vi "generator_set_values.vi"(8 "error in (no error)":errorcluster, 9 "Frequency (1000 Hz)":dbl=1000.0 format="%#.6g", 10 "Amplitude (1.0 Vpp)":dbl=1.0 format="%#.4f", 11 "app_data":T1={"Instruments"={"generator"="", "voltment_with_scaner"="", "voltment_without_scaner"=""}, "boc"={"conParam"={"ReadIntParam"=TRUE, "ReadDescrParam"=FALSE, "ReadFloatParam"=TRUE, "debug"=FALSE, "ReadJSON"=FALSE, "IP_address"="192.168.1.216", "N_attempts"=3, "type_con"=enum."TCP", "MB_address"=1, "VISA"="COM1", "connection ID"=refnum, "nameDevices"="", "timeout"=3000, "port"=2000, "type_version"="0F0C0001", "baud_rate"=115200, "VersionControl"=FALSE, "TCP_conn"=FALSE, "WindowSize"=700}, "Param"={"NumParam"={"NTelem"=0, "NInt"=0, "NFloat"=0, "NTable"=0}, "ParamInt"=[], "Telemetry"=[], "Table"=[], "ParamFloat"=[]}}, "boe"={"conParam"={"ReadIntParam"=TRUE, "ReadDescrParam"=FALSE, "ReadFloatParam"=TRUE, "debug"=FALSE, "ReadJSON"=FALSE, "IP_address"="192.168.1.216", "N_attempts"=3, "type_con"=enum."TCP", "MB_address"=1, "VISA"="COM1", "connection ID"=refnum, "nameDevices"="", "timeout"=3000, "port"=2000, "type_version"="03200100", "baud_rate"=115200, "VersionControl"=FALSE, "TCP_conn"=FALSE, "WindowSize"=700}, "Param"={"NumParam"={"NTelem"=0, "NInt"=0, "NFloat"=0, "NTable"=0}, "ParamInt"=[], "Telemetry"=[], "Table"=[], "ParamFloat"=[]}}, "attenuator_tune_koef"=[]}) -> (0 "error out":errorcluster, 3 "output cluster":T1={"Instruments"={"generator"="", "voltment_with_scaner"="", "voltment_without_scaner"=""}, "boc"={"conParam"={"ReadIntParam"=TRUE, "ReadDescrParam"=FALSE, "ReadFloatParam"=TRUE, "debug"=FALSE, "ReadJSON"=TRUE, "IP_address"="192.168.1.216", "N_attempts"=3, "type_con"=enum."TCP", "MB_address"=1, "VISA"="COM1", "connection ID"=refnum, "nameDevices"="", "timeout"=3000, "port"=2000, "type_version"="0F0C0001", "baud_rate"=115200, "VersionControl"=FALSE, "TCP_conn"=FALSE, "WindowSize"=700}, "Param"={"NumParam"={"NTelem"=0, "NInt"=0, "NFloat"=0, "NTable"=0}, "ParamInt"=[], "Telemetry"=[], "Table"=[], "ParamFloat"=[]}}, "boe"={"conParam"={"ReadIntParam"=TRUE, "ReadDescrParam"=FALSE, "ReadFloatParam"=TRUE, "debug"=FALSE, "ReadJSON"=TRUE, "IP_address"="192.168.1.216", "N_attempts"=3, "type_con"=enum."TCP", "MB_address"=1, "VISA"="COM1", "connection ID"=refnum, "nameDevices"="", "timeout"=3000, "port"=2000, "type_version"="0F0C0001", "baud_rate"=115200, "VersionControl"=FALSE, "TCP_conn"=FALSE, "WindowSize"=700}, "Param"={"NumParam"={"NTelem"=0, "NInt"=0, "NFloat"=0, "NTable"=0}, "ParamInt"=[], "Telemetry"=[], "Table"=[], "ParamFloat"=[]}}, "attenuator_tune_koef"=[]})   [LabVIEW 2017]
uses:
  controls/app_data.ctl
  controls/instruments.ctl
  Unicorn Labview Library/Control/unicorn_Param.ctl
  Unicorn Labview Library/Control/unicorn_conn.ctl
  Unicorn Labview Library/Control/unicorn_JSON.ctl
  Unicorn Labview Library/Control/unicorn_ParamInt.ctl
  Unicorn Labview Library/Control/unicorn_Telemetry.ctl
  Unicorn Labview Library/Control/unicorn_Table.ctl
  Unicorn Labview Library/Control/unicorn_ParamFloat.ctl
  <instrlib>/Siglent SDG X Series/Siglent SDG X Series.lvlib
  Unicorn Labview Library/Unicorn Library.lvlib
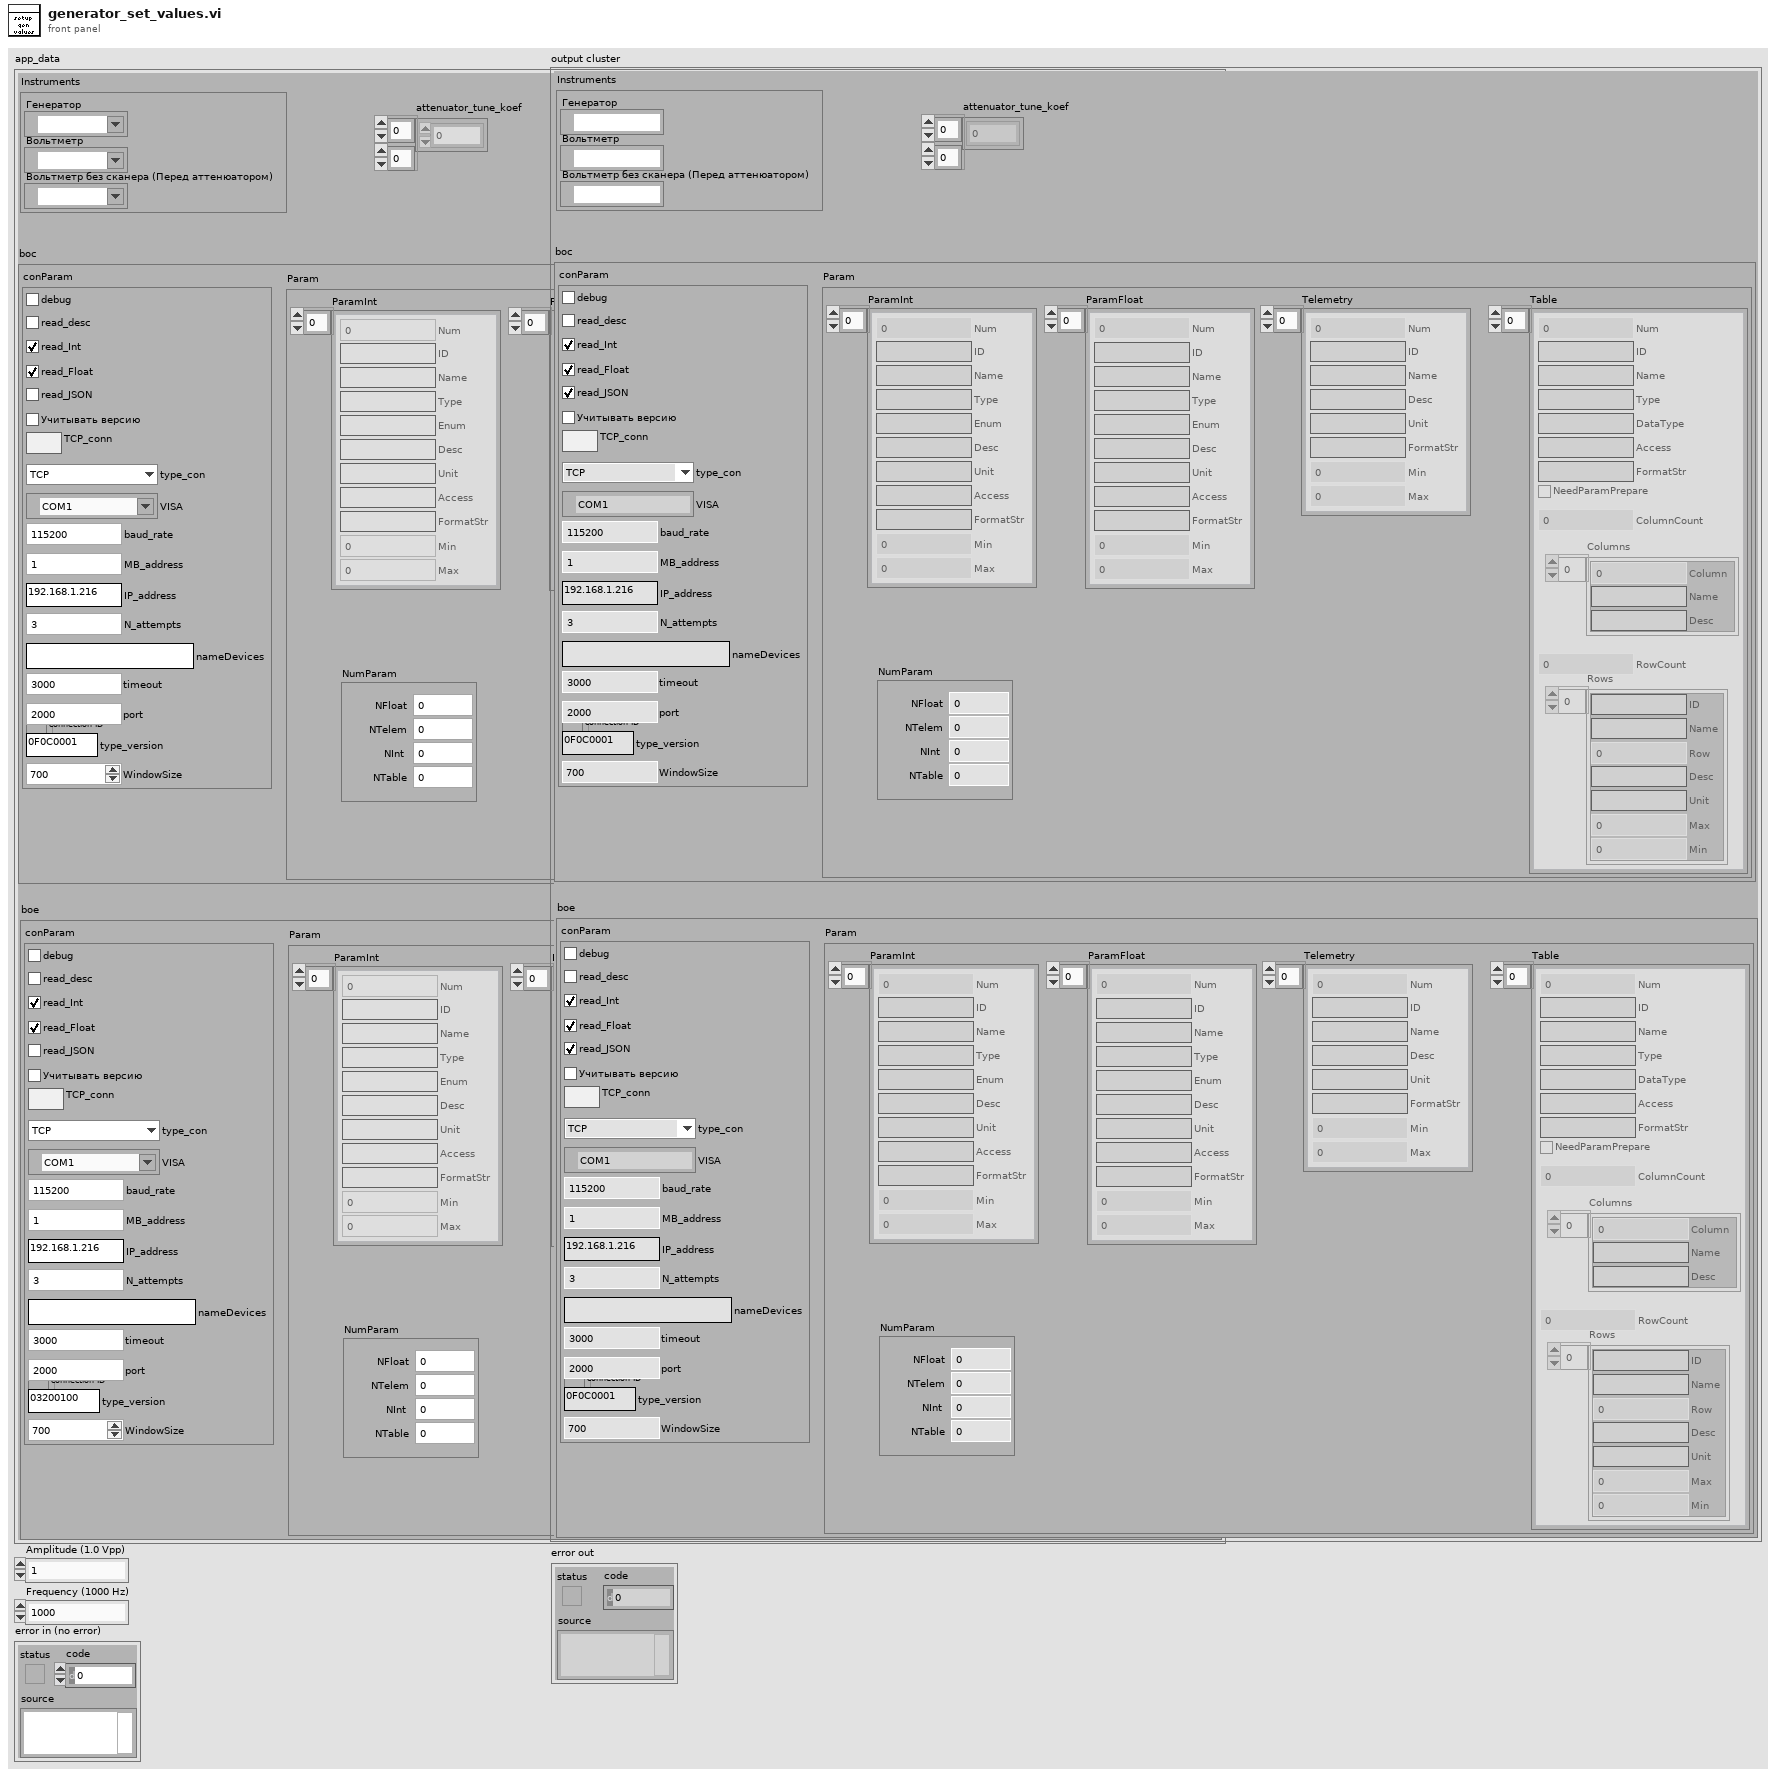
[diagram p1: front panel]
types:
  T1 = typedef "app_data.ctl" = cluster{"Instruments":T2, "boc":T3, "boe":T3, "attenuator_tune_koef":dbl[][]}
  T2 = typedef "instruments.ctl" = cluster{"generator":refnum<visa-resource-name>, "voltment_with_scaner":refnum<visa-resource-name>, "voltment_without_scaner":refnum<visa-resource-name>}
  T3 = typedef "Unicorn Library.lvlib/unicorn_Param.ctl" = cluster{"conParam":T4, "Param":T5}
  T4 = typedef "Unicorn Library.lvlib/unicorn_conn.ctl" = cluster{"ReadIntParam":bool, "ReadDescrParam":bool, "ReadFloatParam":bool, "debug":bool, "ReadJSON":bool, "IP_address":string, "N_attempts":i32, "type_con":enum16{"Serial", "TCP"}, "MB_address":i32, "VISA":refnum<visa-resource-name>, "connection ID":refnum<k5>, "nameDevices":string, "timeout":i32, "port":u16, "type_version":string, "baud_rate":u32, "VersionControl":bool, "TCP_conn":bool, "WindowSize":i32}
  T5 = typedef "Unicorn Library.lvlib/unicorn_JSON.ctl" = cluster{"NumParam":cluster{"NTelem":i32, "NInt":i32, "NFloat":i32, "NTable":i32}, "ParamInt":T6, "Telemetry":T7, "Table":T8, "ParamFloat":T9}
  T6 = typedef "Unicorn Library.lvlib/unicorn_ParamInt.ctl" = cluster{"ID":string, "Num":i32, "Name":string, "Type":string, "Enum":string, "Desc":string, "Unit":string, "Access":string, "FormatStr":string, "Min":i32, "Max":i32}[]
  T7 = typedef "Unicorn Library.lvlib/unicorn_Telemetry.ctl" = cluster{"ID":string, "Num":i32, "Name":string, "Desc":string, "Unit":string, "FormatStr":string, "Min":i32, "Max":i32}[]
  T8 = typedef "Unicorn Library.lvlib/unicorn_Table.ctl" = cluster{"Num":i32, "Access":string, "ColumnCount":i32, "NeedParamPrepare":bool, "Columns":cluster{"Column":i32, "Desc":string, "Name":string}[], "DataType":string, "FormatStr":string, "ID":string, "Name":string, "RowCount":i32, "Rows":cluster{"Desc":string, "ID":string, "Max":i32, "Min":i32, "Name":string, "Row":i32, "Unit":string}[], "Type":string}[]
  T9 = typedef "Unicorn Library.lvlib/unicorn_ParamFloat.ctl" = cluster{"ID":string, "Num":i32, "Name":string, "Type":string, "Enum":string, "Desc":string, "Unit":string, "Access":string, "FormatStr":string, "Min":i32, "Max":i32}[]
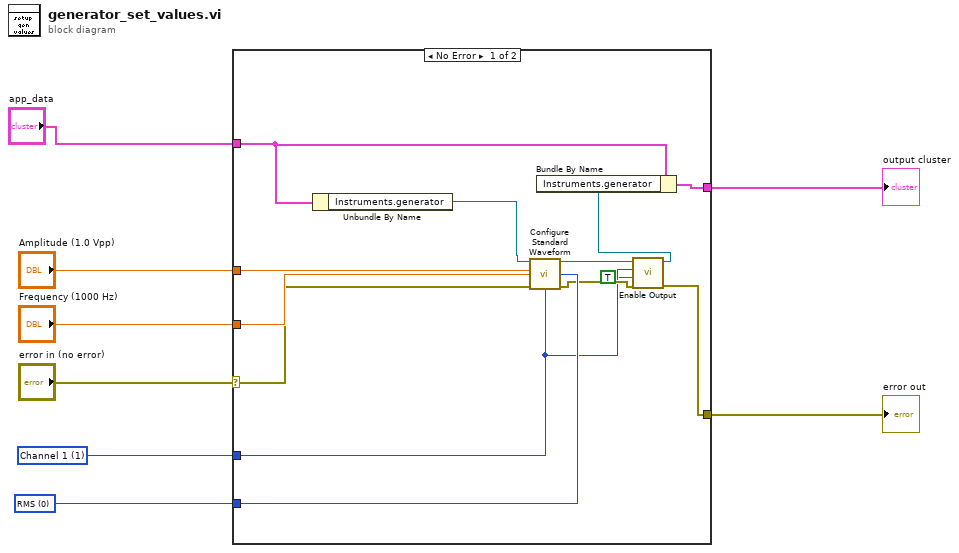
[diagram p0: block diagram]
diagram:
  w7 = 1 items=["Channel 1"=1, "Channel 2"=2] ("Channel (1:Channel 1)")
  w8 = u16 0 items=["RMS", "pp", "dBm"] ("v-type")
  n1 = case shown="No Error" "error in (no error)" {
    selector: "error in (no error)" -> [w15 w22]
    tunnel: w8 -> [w21 _]
    tunnel: w7 -> [w10 _]
    tunnel: "app_data" -> [w19 w23]
    tunnel: "Amplitude (1.0 Vpp)" -> [w18 _]
    tunnel: "Frequency (1000 Hz)" -> [w17 _]
    tunnel: [w13 w22] -> w3
    tunnel: [w16 w23] -> w2
    frame No Error {
      n2 = Unbundle By Name(w19) -> ("Instruments.generator"=w20:refnum<visa-resource-name>)
      n3 = call <instrlib>:"Configure Standard Waveform.vi"("VISA resource name"=w20, "Channel (1:Channel 1)"=w10, "Amplitude (1.0 Vpp)"=w18, "Frequency (1000 Hz)"=w17, "v-type"=w21, "error in (no error)"=w15) -> ("VISA resource name out"=w12:refnum<visa-resource-name>, "error out"=w14:errorcluster)  [unwired: 8 in]
      n4 = call <instrlib>:"Enable Output.vi"("error in (no error)"=w14, "Enable Output (T: Enable)"=TRUE, "Channel (1:Channel 1)"=w10, "VISA resource name"=w12) -> ("error out"=w13:errorcluster, "VISA resource name out"=w11:refnum<visa-resource-name>)  [unwired: 6 in]
      n5 = Bundle By Name(cluster=w19, "Instruments.generator"=w11) -> (w16:T1)
    }
    frame Error {
    }
  }
  "error out" <- w3
  "output cluster" <- w2
